vi "Launch.vi"(10 "Actor":refnum<class "Actor.lvclass">, 11 "Helper Loop in":refnum<class "Helper Loop.lvclass">) -> (0 "error out":errorcluster, 2 "Helper Loop":refnum<class "Helper Loop.lvclass">)   [LabVIEW 2021, in "Helper Loop.lvclass"]
uses:
  Helper Loop.lvclass
  Actor/Actor/Actor.lvclass
  Loop Wrapper.vi
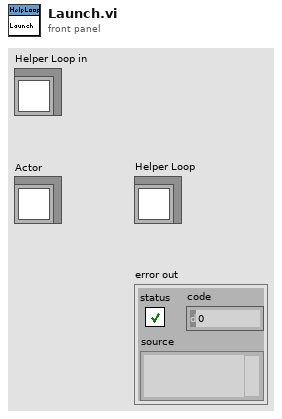
[diagram p1: front panel]
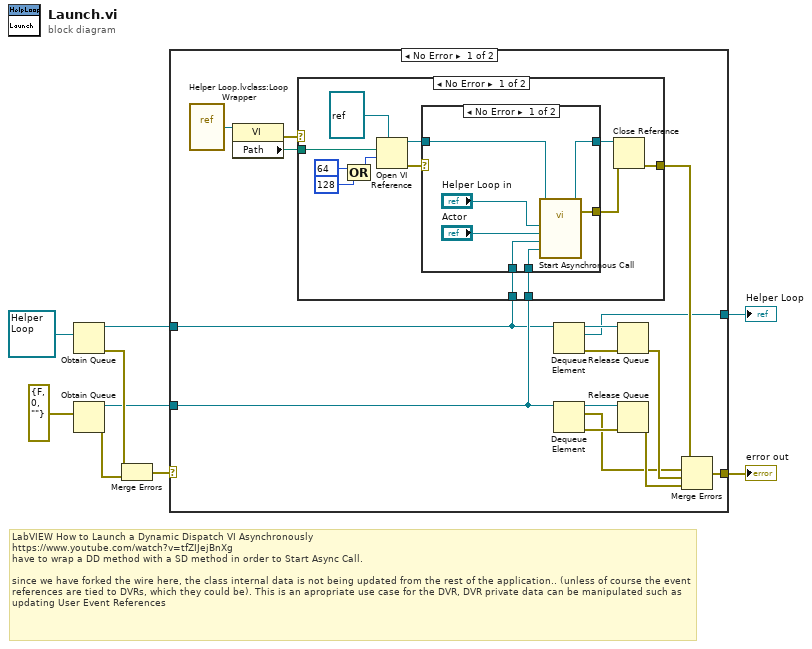
[diagram p0: block diagram]
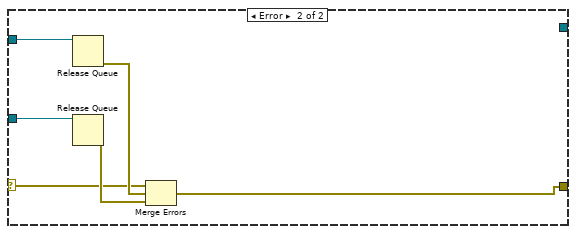
[diagram p4: hidden frame]
diagram:
  # "LabVIEW How to Launch a Dynamic Dispatch VI Asynchronously\nhttps://www.youtube.com/watch?v=tfZIJejBnXg\nhave to wrap a DD method with a SD method in order to Start Async Call.\n\nsince we have forked the wire here, the class internal data is not being updated from the rest of the application.. (unless of course the event references are tied to DVRs, which they could be). This is an apropriate use case for the DVR, DVR private data can be manipulated such as updating User Event References"
  n1 = Obtain Queue(element data type=refnum<class "Helper Loop.lvclass"> refnum ("Helper Loop.lvclass")) -> (queue out=w6:refnum<queue>, error out=w5:errorcluster)  [unwired: 4 in, 1 out]
  n2 = Obtain Queue(element data type=errorcluster {"status"=FALSE, "code"=0, "source"=""} ("error out")) -> (queue out=w1:refnum<queue>, error out=w2:errorcluster)  [unwired: 4 in, 1 out]
  n3 = Merge Errors(w5, w2) -> (w3:errorcluster)
  n4 = case shown="No Error" w3 {
    selector: w3 -> [_ w47]
    tunnel: [w18 _] -> w9
    tunnel: [w20 w51] -> w8
    tunnel: w6 -> [w10 w52]
    tunnel: w1 -> [w17 w49]
    frame No Error {
      n5 = vi-ref "Helper Loop.lvclass:Loop Wrapper.vi"() -> (w22:refnum<vi>)
      n6 = property class="VI"(reference=w22) -> (error out=w23:errorcluster, "Path"=w21:path)  [unwired: 1 in, 1 out]
      n7 = case shown="No Error" w23 {
        selector: w23 -> [_ w46]
        tunnel: [w34 w46] -> w24
        tunnel: w21 -> [w27 _]
        tunnel: w10 -> [w26 _]
        tunnel: w17 -> [w25 _]
        frame No Error {
          n8 = Compound Arithmetic op=OR(64 ("options: Multiple Clones,\n  Fire & Forget"), 128 ("options: Multiple Clones,\n  Fire & Forget")) -> (w32:i32)
          n9 = Open VI Reference(type specifier VI Refnum (for type only)=refnum<vi> refnum, vi path=w27, options=w32) -> (vi reference=w29:refnum<vi>, error out=w30:errorcluster)  [unwired: 3 in]
          n10 = case shown="No Error" w30 {
            selector: w30 -> [_ w45]
            tunnel: [w42 w44] -> w36
            tunnel: [w41 w45] -> w35
            tunnel: w29 -> [w43 w44]
            tunnel: w26 -> [w40 _]
            tunnel: w25 -> [w39 _]
            frame No Error {
              n11 = call-by-ref "Start Asynchronous Call"(reference=w43, "Error Q"=w39, "Helper Loop Q"=w40, "Actor"="Actor", "Helper Loop in"="Helper Loop in") -> (reference out=w42:refnum<vi>, error out=w41:errorcluster)  [unwired: 9 in]
            }
            frame Error {
            }
          }
          n12 = Close Reference(reference=w36, error in (no error)=w35) -> (error out=w34:errorcluster)
        }
        frame Error {
        }
      }
      n13 = Dequeue Element(queue=w10) -> (queue out=w19:refnum<queue>, element=w18:refnum<class "Helper Loop.lvclass">, error out=w15:errorcluster)  [unwired: 2 in, 1 out]
      n14 = Dequeue Element(queue=w17) -> (queue out=w16:refnum<queue>, element=w11:errorcluster, error out=w13:errorcluster)  [unwired: 2 in, 1 out]
      n15 = Release Queue(queue=w19, error in (no error)=w15) -> (error out=w14:errorcluster)  [unwired: 1 in, 2 out]
      n16 = Release Queue(queue=w16, error in (no error)=w13) -> (error out=w12:errorcluster)  [unwired: 1 in, 2 out]
      n17 = Merge Errors(w24, w11, w14, w12) -> (w20:errorcluster)
    }
    frame Error {
      n18 = Release Queue(queue=w52) -> (error out=w50:errorcluster)  [unwired: 2 in, 2 out]
      n19 = Release Queue(queue=w49) -> (error out=w48:errorcluster)  [unwired: 2 in, 2 out]
      n20 = Merge Errors(w47, w50, w48) -> (w51:errorcluster)
    }
  }
  "error out" <- w8
  "Helper Loop" <- w9
